vi "Query Remote Trace Log Contents.vi"(7 "Start (1)":i32=1, 8 "error in (no error)":errorcluster, 9 "Count (1)":i32=1, 10 "Rows (Latest)":i32(ring) items=["Latest", "List", "Error", "Connection"], 11 "VISA resource name":refnum<visa-resource-name>) -> (0 "error out":errorcluster, 2 "Log":string, 3 "VISA resource name out":refnum<visa-resource-name>)   [LabVIEW 2020, in "Rohde&Schwarz CMXP Base.lvlib"]
doc: "Queries the contents of the remote trace log.\n\nAttribute:\nRSCMXPBASE_ATTR_REMOTE_TRACE_LOG_CONTENTS\n\nRemote-control command:\nFETCh:BASE:RTRace:ROWS?"
uses:
  <instrlib>/Rohde&Schwarz CMXP Base/Rohde&Schwarz CMXP Base.lvlib
  <instrlib>/Rohde&Schwarz CMXP Base/Private/rsidr_core.llb/rsidr_core.lvlib
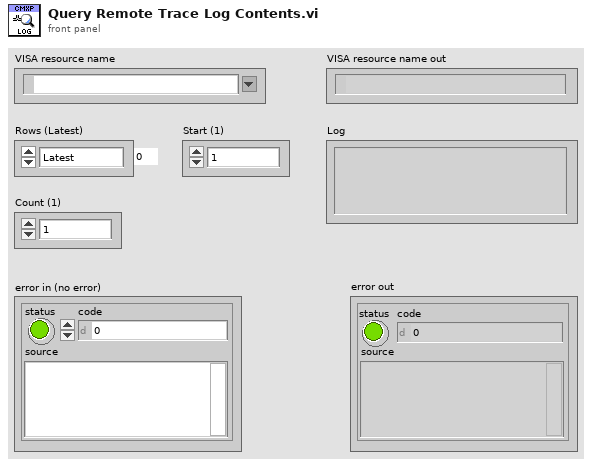
[diagram p1: front panel]
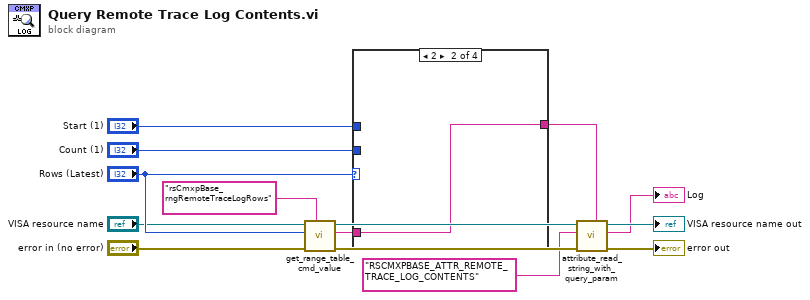
[diagram p0: block diagram]
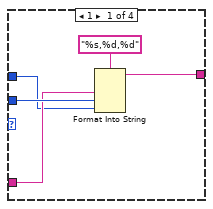
[diagram p2: hidden frame]
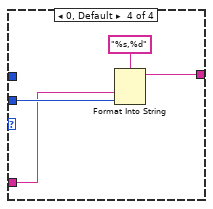
[diagram p4: hidden frame]
diagram:
  n1 = call <instrlib>:"get_range_table_cmd_value.vi"("Range Table ID in"="rsCmxpBase_rngRemoteTraceLogRows", "error in"="error in (no error)", "Input Int32 value"="Rows (Latest)", "VISA resource name"="VISA resource name") -> ("error out"=w11:errorcluster, "Cmd value out"=w10:string, "VISA resource name out"=w12:refnum<visa-resource-name>)  [unwired: 5 in]
  n2 = case shown="2" "Rows (Latest)" {
    tunnel: w10 -> [w16 w20 w21 w22]
    tunnel: "Count (1)" -> [w18 _ _ w24]
    tunnel: [w17 w20 w21 w23] -> w6
    tunnel: "Start (1)" -> [w15 _ _ _]
    frame 1 {
      n3 = Format Into String(format string="%s,%d,%d", w16, w18, w15) -> (resulting string=w17:string)  [unwired: 2 in, 1 out]
    }
    frame 2 {
    }
    frame 3 {
    }
    frame 0, Default {
      n4 = Format Into String(format string="%s,%d", w22, w24) -> (resulting string=w23:string)  [unwired: 2 in, 1 out]
    }
  }
  n5 = call <instrlib>:"attribute_read_string_with_query_param.vi"("Query Parameter (None)"=w6, "error in"=w11, "Attribute ID"="RSCMXPBASE_ATTR_REMOTE_TRACE_LOG_CONTENTS", "VISA resource name"=w12) -> ("error out"=→"error out":errorcluster, "String out"=→"Log":string, "VISA resource name out"=→"VISA resource name out":refnum<visa-resource-name>)  [unwired: 5 in]
